vi "SIM_Flow.vi"() -> (1 "Flow (ml/min)":dbl format="%.2f")   [LabVIEW 2016]
panel:
  in  "Static value":dbl=10.0 format="%.2f"
  in  "Static":bool
  in  "sim_high":dbl=20.0 format="%.2f"
  in  "sim_low":dbl=15.0 format="%.2f"
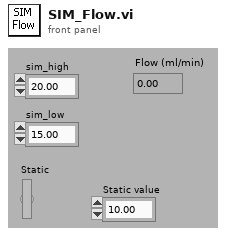
[diagram p1: front panel]
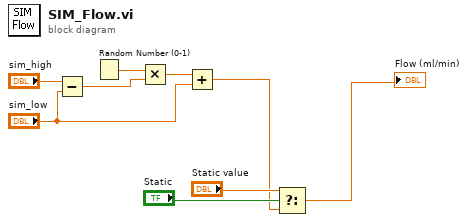
[diagram p0: block diagram]
diagram:
  n1 = Subtract(x="sim_high", y="sim_low") -> (x-y=w7:dbl)
  n2 = Random Number (0-1)() -> (number: 0 to 1=w8:dbl)
  n3 = Multiply(x=w8, y=w7) -> (x*y=w6:dbl)
  n4 = Add(x=w6, y="sim_low") -> (x+y=w2:dbl)
  n5 = Select(t="Static value", s="Static", f=w2) -> (s? t:f=→"Flow (ml/min)":dbl)
